vi "AbsEncPos_Get.vi"(11 "Update?":bool) -> (0 "RearRightPulsePos":i32, 1 "RearLeftPulsePos":i32, 2 "FrontRightPulsePos":i32, 3 "FrontLeftPulsePos":i32)   [LabVIEW 2018]
uses:
  <vilib>/Rock Robotics/WPI/ThirdParty/Phoenix-LabVIEW/Motor Controller/Get/CTRE_Phoenix_MotorController_GetPulseWidthAll.vi
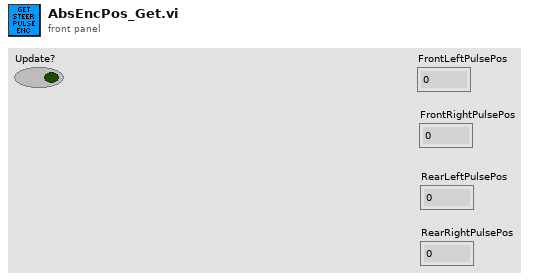
[diagram p1: front panel]
types:
  T1 = typedef "WPI_MotorControlDeviceRef.ctl" = cluster{"DeviceStatus":errorcluster, "Type":T2, "PWM":cluster{"PWM Channel":T3, "DeadBand":T4}, "CAN":cluster{"Device Number":u8, "SetOutput VI Ref":variant, "GetOutput VI Ref":variant, "Enable VI Ref":variant, "Disable VI Ref":variant, "Data":variant}, "Invert":bool, "DIO PWM":cluster{"PWM \"Enable\" Channel":T3, "DIOChannel":T5, "PWM Rate":dbl}}
  T2 = typedef "WPI_MotorControlType.ctl" = enum16{"PWM", "CAN", "DIO PWM"}
  T3 = typedef "FPGA_DIOPWMChannel.ctl" = enum8{"PWM 0", "PWM 1", "PWM 2", "PWM 3", "PWM 4", "PWM 5", "PWM 6", "PWM 7", "PWM 8", "PWM 9", "PWM MXP 0", "PWM MXP 1", "PWM MXP 2", "PWM MXP 3", "PWM MXP 4", "PWM MXP 5", "PWM MXP 6", "PWM MXP 7", "PWM MXP 8", "PWM MXP 9", "Invalid"}
  T4 = typedef "WPI_PWMDeadband.ctl" = cluster{"Name":string, "maxPositivePwm":i32, "minPositivePwm":i32, "centerPwm":i32, "maxNegativePwm":i32, "minNegativePwm":i32, "angularRange":u16}
  T5 = typedef "FPGA_DIOChannel.ctl" = enum8{"DIO 0", "DIO 1", "DIO 2", "DIO 3", "DIO 4", "DIO 5", "DIO 6", "DIO 7", "DIO 8", "DIO 9", "DIO MXP 0", "DIO MXP 1", "DIO MXP 2", "DIO MXP 3", "DIO MXP 4", "DIO MXP 5", "DIO MXP 6", "DIO MXP 7", "DIO MXP 8", "DIO MXP 9", "DIO MXP 10", "DIO MXP 11", "DIO MXP 12", "DIO MXP 13", "DIO MXP 14", "DIO MXP 15", "SPI Port CS1", "SPI Port CS2", "SPI Port CS3", "SPI Port MISO", "SPI Port MOSI", "Invalid"}
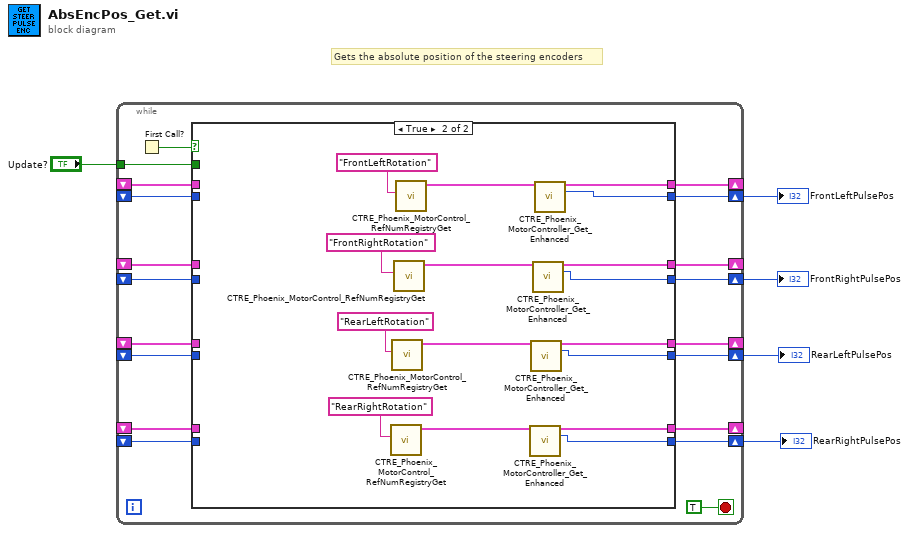
[diagram p0: block diagram]
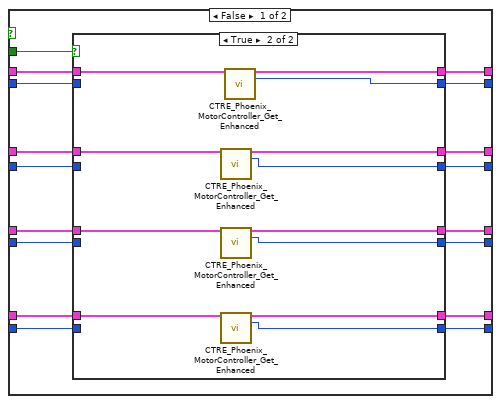
[diagram p2: hidden frame]
diagram:
  # "Gets the absolute position of the steering encoders"
  n1 = while {
    shift-right: [w23] -> _
    shift-left: _ -> [w22]
    tunnel: "Update?" -> [w20]
    shift-right: [w24] -> w5
    shift-left: _ -> [w19]
    shift-right: [w18] -> _
    shift-left: _ -> [w12]
    shift-right: [w17] -> w1
    shift-left: _ -> [w9]
    shift-right: [w16] -> _
    shift-left: _ -> [w11]
    shift-right: [w15] -> w2
    shift-left: _ -> [w8]
    shift-right: [w14] -> _
    shift-left: _ -> [w10]
    shift-right: [w13] -> w3
    shift-left: _ -> [w7]
    stop <- TRUE stop-if-true
    n2 = First Call?() -> (First Call?: T/F=w21:bool)
    n3 = case shown="True" w21 {
      tunnel: w22 -> [w41 _]
      tunnel: [w40 w74] -> w24
      tunnel: [w39 w75] -> w23
      tunnel: w20 -> [w38 _]
      tunnel: w19 -> [w37 _]
      tunnel: [w35 w67] -> w18
      tunnel: [w30 w66] -> w17
      tunnel: [w34 w65] -> w16
      tunnel: [w29 w64] -> w15
      tunnel: [w31 w63] -> w14
      tunnel: [w28 w62] -> w13
      tunnel: w12 -> [w36 _]
      tunnel: w11 -> [w33 _]
      tunnel: w10 -> [w32 _]
      tunnel: w9 -> [w27 _]
      tunnel: w8 -> [w26 _]
      tunnel: w7 -> [w25 _]
      frame False {
        n4 = case shown="True" w38 {
          tunnel: w41 -> [w49 w61]
          tunnel: [w48 w60] -> w40
          tunnel: [w49 w59] -> w39
          tunnel: w37 -> [w48 _]
          tunnel: w36 -> [w47 w58]
          tunnel: [w47 w57] -> w35
          tunnel: [w46 w56] -> w34
          tunnel: w33 -> [w46 w55]
          tunnel: w32 -> [w45 w54]
          tunnel: [w45 w53] -> w31
          tunnel: [w44 w52] -> w30
          tunnel: [w43 w51] -> w29
          tunnel: [w42 w50] -> w28
          tunnel: w27 -> [w44 _]
          tunnel: w26 -> [w43 _]
          tunnel: w25 -> [w42 _]
          frame False {
          }
          frame True {
            n5 = call-poly <vilib>:"CTRE_Phoenix_MotorController_Get_Enhanced.vi"("PhoenixMotorControlDevRef"=w58) -> ("PhoenixMotorControlDevRef"=w57:T1, "Pulse Width Position"=w52:i32)  [unwired: 9 in, 4 out]
            n6 = call-poly <vilib>:"CTRE_Phoenix_MotorController_Get_Enhanced.vi"("PhoenixMotorControlDevRef"=w55) -> ("PhoenixMotorControlDevRef"=w56:T1, "Pulse Width Position"=w51:i32)  [unwired: 9 in, 4 out]
            n7 = call-poly <vilib>:"CTRE_Phoenix_MotorController_Get_Enhanced.vi"("PhoenixMotorControlDevRef"=w54) -> ("PhoenixMotorControlDevRef"=w53:T1, "Pulse Width Position"=w50:i32)  [unwired: 9 in, 4 out]
            n8 = call-poly <vilib>:"CTRE_Phoenix_MotorController_Get_Enhanced.vi"("PhoenixMotorControlDevRef"=w61) -> ("PhoenixMotorControlDevRef"=w59:T1, "Pulse Width Position"=w60:i32)  [unwired: 9 in, 4 out]
          }
        }
      }
      frame True {
        n9 = call <vilib>:"CTRE_Phoenix_MotorControl_RefNumRegistryGet.vi"("refnum name"="RearRightRotation") -> ("PhoenixMotorControlDevRef"=w69:T1)  [unwired: 9 in, 1 out]
        n10 = call <vilib>:"CTRE_Phoenix_MotorControl_RefNumRegistryGet.vi"("refnum name"="RearLeftRotation") -> ("PhoenixMotorControlDevRef"=w70:T1)  [unwired: 9 in, 1 out]
        n11 = call <vilib>:"CTRE_Phoenix_MotorControl_RefNumRegistryGet.vi"("refnum name"="FrontRightRotation") -> ("PhoenixMotorControlDevRef"=w73:T1)  [unwired: 9 in, 1 out]
        n12 = call <vilib>:"CTRE_Phoenix_MotorControl_RefNumRegistryGet.vi"("refnum name"="FrontLeftRotation") -> ("PhoenixMotorControlDevRef"=w76:T1)  [unwired: 9 in, 1 out]
        n13 = call-poly <vilib>:"CTRE_Phoenix_MotorController_Get_Enhanced.vi"("PhoenixMotorControlDevRef"=w69) -> ("PhoenixMotorControlDevRef"=w63:T1, "Pulse Width Position"=w62:i32)  [unwired: 9 in, 4 out]
        n14 = call-poly <vilib>:"CTRE_Phoenix_MotorController_Get_Enhanced.vi"("PhoenixMotorControlDevRef"=w70) -> ("PhoenixMotorControlDevRef"=w65:T1, "Pulse Width Position"=w64:i32)  [unwired: 9 in, 4 out]
        n15 = call-poly <vilib>:"CTRE_Phoenix_MotorController_Get_Enhanced.vi"("PhoenixMotorControlDevRef"=w73) -> ("PhoenixMotorControlDevRef"=w67:T1, "Pulse Width Position"=w66:i32)  [unwired: 9 in, 4 out]
        n16 = call-poly <vilib>:"CTRE_Phoenix_MotorController_Get_Enhanced.vi"("PhoenixMotorControlDevRef"=w76) -> ("PhoenixMotorControlDevRef"=w75:T1, "Pulse Width Position"=w74:i32)  [unwired: 9 in, 4 out]
      }
    }
  }
  "FrontLeftPulsePos" <- w5
  "FrontRightPulsePos" <- w1
  "RearLeftPulsePos" <- w2
  "RearRightPulsePos" <- w3
